vi "Brosse.vi"(0 "lift brosse":bool, 1 "brosse":bool) -> ()   [LabVIEW 2017]
uses:
  <vilib>/Rock Robotics/WPI/ThirdParty/Phoenix-LabVIEW/Motor Controller/Controls/CTRE_Phoenix_MotorControl_ControlMode.ctl
  <vilib>/Rock Robotics/WPI/DriverStation/WPI_DriverStationRobotMode2.ctl
  Robot Global Data.vi
  <vilib>/Rock Robotics/Network Tables/NT Write Boolean.vi
panel:
  out "Distance":dbl
  in  "dist haut":dbl
  in  "dist bas":dbl
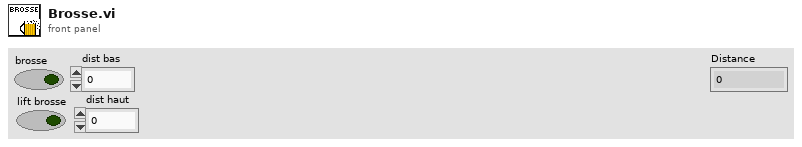
[diagram p1: front panel]
types:
  T1 = typedef "WPI_DriverStationRobotMode2.ctl" = enum16{"Autonomous Disabled", "Autonomous Enabled", "Teleop Disabled", "Teleop Enabled", "Disconnected", "Finish", "Test Disabled", "Test Enabled", "Emergency Stopped"}
  T2 = typedef "CTRE_Phoenix_MotorControl_ControlMode.ctl" = u16
  T3 = typedef "WPI_MotorControlDeviceRef.ctl" = cluster{"DeviceStatus":errorcluster, "Type":T4, "PWM":cluster{"PWM Channel":T5, "DeadBand":T6}, "CAN":cluster{"Device Number":u8, "SetOutput VI Ref":variant, "GetOutput VI Ref":variant, "Enable VI Ref":variant, "Disable VI Ref":variant, "Data":variant}, "Invert":bool, "DIO PWM":cluster{"PWM \"Enable\" Channel":T5, "DIOChannel":T7, "PWM Rate":dbl}}
  T4 = typedef "WPI_MotorControlType.ctl" = enum16{"PWM", "CAN", "DIO PWM"}
  T5 = typedef "FPGA_DIOPWMChannel.ctl" = enum8{"PWM 0", "PWM 1", "PWM 2", "PWM 3", "PWM 4", "PWM 5", "PWM 6", "PWM 7", "PWM 8", "PWM 9", "PWM MXP 0", "PWM MXP 1", "PWM MXP 2", "PWM MXP 3", "PWM MXP 4", "PWM MXP 5", "PWM MXP 6", "PWM MXP 7", "PWM MXP 8", "PWM MXP 9", "Invalid"}
  T6 = typedef "WPI_PWMDeadband.ctl" = cluster{"Name":string, "maxPositivePwm":i32, "minPositivePwm":i32, "centerPwm":i32, "maxNegativePwm":i32, "minNegativePwm":i32, "angularRange":u16}
  T7 = typedef "FPGA_DIOChannel.ctl" = enum8{"DIO 0", "DIO 1", "DIO 2", "DIO 3", "DIO 4", "DIO 5", "DIO 6", "DIO 7", "DIO 8", "DIO 9", "DIO MXP 0", "DIO MXP 1", "DIO MXP 2", "DIO MXP 3", "DIO MXP 4", "DIO MXP 5", "DIO MXP 6", "DIO MXP 7", "DIO MXP 8", "DIO MXP 9", "DIO MXP 10", "DIO MXP 11", "DIO MXP 12", "DIO MXP 13", "DIO MXP 14", "DIO MXP 15", "SPI Port CS1", "SPI Port CS2", "SPI Port CS3", "SPI Port MISO", "SPI Port MOSI", "Invalid"}
  T8 = typedef "WPI_EncoderDevRef.ctl" = cluster{"DevStatus":errorcluster, "EncoderIndex":T9, "CounterIndex":T10, "DistancePerCount":dbl, "Decoding Type":T11}
  T9 = typedef "FPGA_EncoderIdx.ctl" = enum8{"Enc 0", "Enc 1", "Enc 2", "Enc 3", "Enc 4", "Enc 5", "Enc 6", "Enc 7", "Invalid"}
  T10 = typedef "FPGA_CounterCtrSystemIndex.ctl" = enum8{"Ctr 0", "Ctr 1", "Ctr 2", "Ctr 3", "Ctr 4", "Ctr 5", "Ctr 6", "Ctr 7", "Invalid"}
  T11 = typedef "WPI_EncoderType.ctl" = enum16{"1x", "2x", "4x"}
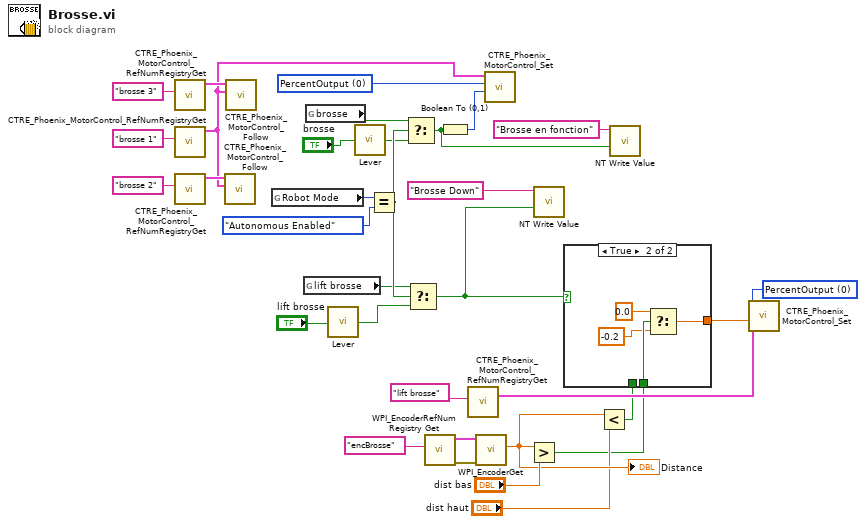
[diagram p0: block diagram]
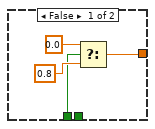
[diagram p2: hidden frame]
diagram:
  w24 = T2 0 items=["PercentOutput"=0, "Position"=1, "Velocity"=2, "Current"=3, "Follower"=5, "MotionProfile"=6, "MotionMagic"=7, "MotionMagicArc"=8, "MotionProfileArc"=10, "Disabled"=15] ("Control Mode")
  w25 = T2 0 items=["PercentOutput"=0, "Position"=1, "Velocity"=2, "Current"=3, "Follower"=5, "MotionProfile"=6, "MotionMagic"=7, "MotionMagicArc"=8, "MotionProfileArc"=10, "Disabled"=15] ("Control Mode")
  n1 = call <vilib>:"CTRE_Phoenix_MotorControl_RefNumRegistryGet.vi"("refnum name"="brosse 3") -> ("PhoenixMotorControlDevRef"=w28:T3)  [unwired: 9 in, 1 out]
  n2 = call <vilib>:"CTRE_Phoenix_MotorControl_RefNumRegistryGet.vi"("refnum name"="brosse 1") -> ("PhoenixMotorControlDevRef"=w26:T3)  [unwired: 9 in, 1 out]
  n3 = call <vilib>:"CTRE_Phoenix_MotorControl_RefNumRegistryGet.vi"("refnum name"="brosse 2") -> ("PhoenixMotorControlDevRef"=w27:T3)  [unwired: 9 in, 1 out]
  n4 = call <vilib>:"CTRE_Phoenix_MotorControl_Follow.vi"("Master Controller to Follow"=w26, "PhoenixMotorControlDevRef"=w27) -> ()  [unwired: 8 in, 2 out]
  n5 = call <vilib>:"CTRE_Phoenix_MotorControl_Follow.vi"("Master Controller to Follow"=w26, "PhoenixMotorControlDevRef"=w28) -> ()  [unwired: 8 in, 2 out]
  n6 = global read "Robot Global Data.vi" "Robot Mode"() -> (w23:T1)
  n7 = global read "Robot Global Data.vi" "lift brosse"() -> (w19:bool)
  n8 = global read "Robot Global Data.vi" "brosse"() -> (w20:bool)
  n9 = call "Lever.vi"("Input"="lift brosse") -> ("Output"=w13:bool)
  n10 = call "Lever.vi"("Input"="brosse") -> ("Output"=w11:bool)
  n11 = Equal?(x=w23, y=WPI_DriverStationRobotMode2."Autonomous Enabled" ("Robot Mode")) -> (x = y?=w21:bool)
  n12 = Select(t=w20, s=w21, f=w11) -> (s? t:f=w4:bool)
  n13 = Select(t=w19, s=w21, f=w13) -> (s? t:f=w2:bool)
  n14 = call <vilib>:"WPI_EncoderRefNum Registry Get.vi"("refnum name"="encBrosse") -> ("error out"=w17:errorcluster, "EncoderDevRef"=w16:T8)  [unwired: 9 in]
  n15 = Boolean To (0,1)(Boolean=w4) -> (0, 1=w18:i16)
  n16 = call <vilib>:"CTRE_Phoenix_MotorControl_RefNumRegistryGet.vi"("refnum name"="lift brosse") -> ("PhoenixMotorControlDevRef"=w33:T3)  [unwired: 9 in, 1 out]
  n17 = call <vilib>:"WPI_EncoderGet.vi"("error in (no error)"=w17, "EncoderDevRef"=w16) -> ("Distance"=w9:dbl)  [unwired: 4 in, 5 out]
  "Distance" <- w9
  n18 = call <vilib>:"CTRE_Phoenix_MotorControl_Set.vi"("Output"=w18, "Control Mode"=w25, "PhoenixMotorControlDevRef"=w26) -> ()  [unwired: 7 in, 2 out]
  n19 = Greater?(x=w9, y="dist bas") -> (0:w7:bool)
  n20 = call-poly <vilib>:"NT Write Value.vi"("Boolean"=w2, "Name"="Brosse Down") -> ()  [unwired: 9 in, 1 out]
  n21 = Less?(x=w9, y="dist haut") -> (x < y?=w5:bool)
  n22 = case shown="True" w2 {
    tunnel: w7 -> [_ w41]
    tunnel: [w37 w38] -> w6
    tunnel: w5 -> [w35 _]
    frame False {
      n23 = Select(t=0.0, s=w35, f=0.8) -> (s? t:f=w37:dbl)
    }
    frame True {
      n24 = Select(t=0.0, s=w41, f=-0.2 ("t")) -> (s? t:f=w38:dbl)
    }
  }
  n25 = call-poly <vilib>:"NT Write Value.vi"("Boolean"=w4, "Name"="Brosse en fonction") -> ()  [unwired: 9 in, 1 out]
  n26 = call <vilib>:"CTRE_Phoenix_MotorControl_Set.vi"("Output"=w6, "Control Mode"=w24, "PhoenixMotorControlDevRef"=w33) -> ()  [unwired: 7 in, 2 out]
